vi "R3_AR pH Control.vi"(8 "Pump On Time (s)":dbl=7.0, 9 "Reaction Time (s)":dbl=7.0, 10 "pH Set Point":dbl=7.0, 11 "pH Tolerance":dbl=20.0) -> ()   [LabVIEW 2016]
uses:
  R3 Reactor Status v1.ctl
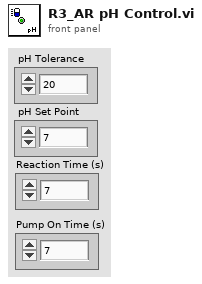
[diagram p1: front panel]
types:
  T1 = cluster{"AR Acid Pump":bool, "AR Base Pump":bool}
  T2 = typedef "R3Variables.lvlib/R3 Reactor Status v1.ctl" = cluster{"AR  Influent":bool, "AR Effluent":bool, "PR Acid":bool, "PR Base":bool, "Feed":bool, "Aeration":bool, "Decant":bool, "pH 1":dbl, "DO (mg/L)":dbl, "pH 1 Amp (A)":dbl, "DO Amp (A)":dbl, "Recycle":bool, "Stirring":bool, "Reactor Status":dbl, "AR Acid":bool, "AR Base":bool, "pH 2":dbl, "pH 2 Amp (A)":dbl}
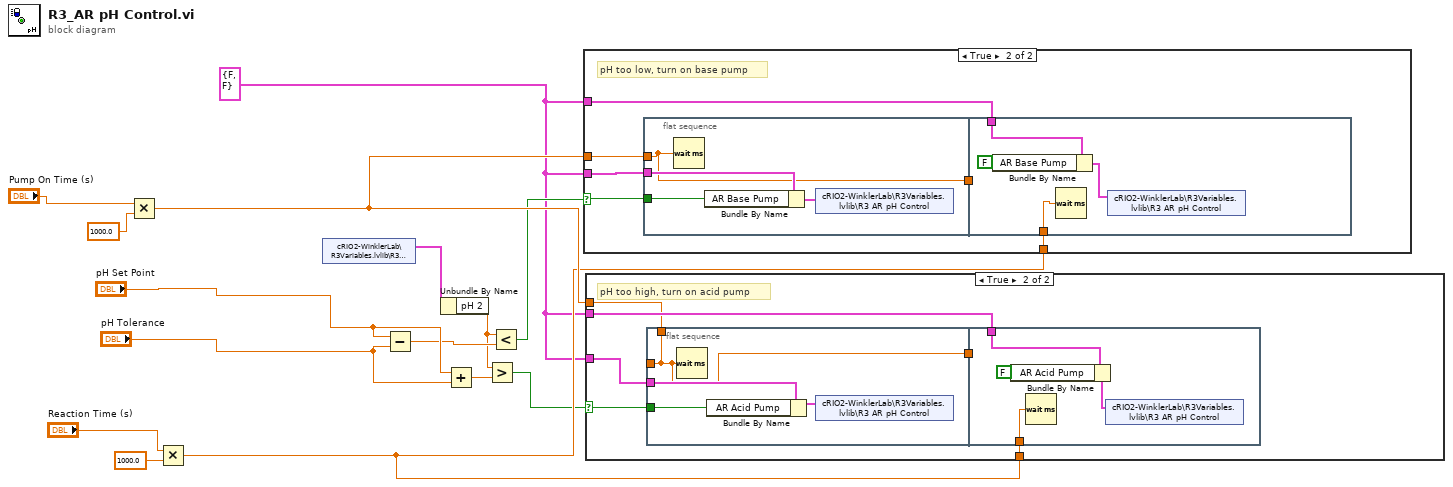
[diagram p0: block diagram]
diagram:
  w1 = T1 {"AR Acid Pump"=FALSE, "AR Base Pump"=FALSE} ("Reactor 3 pH Control-2")
  n1 = Multiply(x="Pump On Time (s)", y=1000.0) -> (x*y=w9:dbl)
  n2 = Multiply(x="Reaction Time (s)", y=1000.0) -> (x*y=w8:dbl)
  n3 = shared-variable "cRIO2-WinklerLab\\R3Variables.lvlib\\R3 Status"() -> (w2:T2)  [unwired: 1 in, 1 out]
  n4 = Subtract(x="pH Set Point", y="pH Tolerance") -> (x-y=w6:dbl)
  n5 = Unbundle By Name(w2) -> ("pH 2"=w4:dbl)
  n6 = Add(x="pH Set Point", y="pH Tolerance") -> (x+y=w7:dbl)
  n7 = Greater?(x=w4, y=w7) -> (0:w3:bool)
  n8 = Less?(x=w4, y=w6) -> (x < y?=w5:bool)
  n9 = case shown="True" w5 {
    selector: w5 -> [_ w21]
    tunnel: w1 -> [_ w20]
    tunnel: w1 -> [_ w19]
    tunnel: w9 -> [_ w17]
    tunnel: w8 -> [_ w16]
    frame False {
    }
    frame True {
      # "pH too low, turn on base pump"
      n10 = flat-sequence {
        tunnel: w21 -> [w24]
        tunnel: w20 -> [w25]
        tunnel: [w22] -> w18
        tunnel: w17 -> [w22]
        tunnel: w19 -> [w29]
        tunnel: w18 -> [_]
        tunnel: w16 -> [w26]
        frame #0 {
          n11 = Wait (ms)(milliseconds to wait=w22) -> ()  [unwired: 1 out]
          n12 = Bundle By Name(cluster=w25, "AR Base Pump"=w24) -> (w23:T1)
          n13 = shared-variable "cRIO2-WinklerLab\\R3Variables.lvlib\\R3 AR pH Control"(w23) -> ()  [unwired: 1 in, 1 out]
        }
        frame #1 {
          n14 = Bundle By Name(cluster=w29, "AR Base Pump"=FALSE ("On/Off")) -> (w27:T1)
          n15 = Wait (ms)(milliseconds to wait=w26) -> ()  [unwired: 1 out]
          n16 = shared-variable "cRIO2-WinklerLab\\R3Variables.lvlib\\R3 AR pH Control"(w27) -> ()  [unwired: 1 in, 1 out]
        }
      }
    }
  }
  n17 = case shown="True" w3 {
    selector: w3 -> [_ w35]
    tunnel: w1 -> [_ w34]
    tunnel: w1 -> [_ w33]
    tunnel: w9 -> [_ w31]
    tunnel: w8 -> [_ w30]
    frame False {
    }
    frame True {
      # "pH too high, turn on acid pump"
      n18 = flat-sequence {
        tunnel: w35 -> [w39]
        tunnel: [w36] -> _
        tunnel: w34 -> [w38]
        tunnel: [w36] -> w32
        tunnel: w31 -> [w36]
        tunnel: w33 -> [w42]
        tunnel: w32 -> [_]
        tunnel: w30 -> [w40]
        frame #0 {
          n19 = Wait (ms)(milliseconds to wait=w36) -> ()  [unwired: 1 out]
          n20 = Bundle By Name(cluster=w38, "AR Acid Pump"=w39) -> (w37:T1)
          n21 = shared-variable "cRIO2-WinklerLab\\R3Variables.lvlib\\R3 AR pH Control"(w37) -> ()  [unwired: 1 in, 1 out]
        }
        frame #1 {
          n22 = Bundle By Name(cluster=w42, "AR Acid Pump"=FALSE ("On/Off")) -> (w41:T1)
          n23 = Wait (ms)(milliseconds to wait=w40) -> ()  [unwired: 1 out]
          n24 = shared-variable "cRIO2-WinklerLab\\R3Variables.lvlib\\R3 AR pH Control"(w41) -> ()  [unwired: 1 in, 1 out]
        }
      }
    }
  }
